vi "createNewExcelDocument.vi"(8 "error in (no error)":errorcluster, 10 "Excel File Path":path, 11 "workbook in":refnum<class "workbook.lvclass">) -> (0 "error out":errorcluster, 3 "workbook out":refnum<class "workbook.lvclass">)   [LabVIEW 2017, in "Excel_Specific.lvlib" / "workbook.lvclass"]
uses:
  workbook.lvclass
  C:/Users/Neo/Desktop/Dev_Tools_BR/LabVIEW_NPOI/src/lib/NPOI 2.1.1/NPOI.OOXML.dll
  lib/NPOI 2.1.1/NPOI.OOXML.dll
  workbook.lvclass/workbook.ctl
  worksheet/worksheet.lvclass
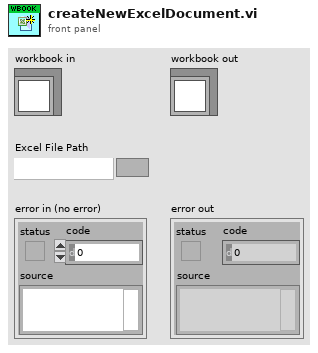
[diagram p1: front panel]
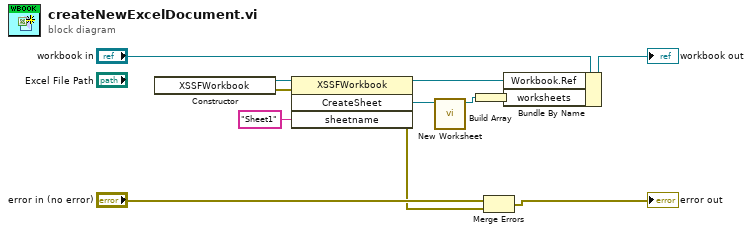
[diagram p0: block diagram]
diagram:
  n1 = constructor class="XSSFWorkbook"() -> (reference out=w9:refnum<k24>, error out=w10:errorcluster)  [unwired: 3 in, 1 out]
  n2 = invoke class="XSSFWorkbook" method="CreateSheet"(reference=w9, error in=w10, "sheetname"="Sheet1") -> (reference out=w6:refnum<k24>, error out=w4:errorcluster, "CreateSheet"=w3:refnum<k24>)  [unwired: 1 in, 1 out]
  n3 = call "New Worksheet.vi"("Worksheet.Ref"=w3) -> ("worksheet out"=w2:refnum<class "worksheet.lvclass">)  [unwired: 9 in, 1 out]
  n4 = Build Array(w2) -> (w1:refnum<class "worksheet.lvclass">[])
  n5 = Merge Errors("error in (no error)", w4) -> (→"error out":errorcluster)
  n6 = Bundle By Name(cluster="workbook in", "Workbook.Ref"=w6, "worksheets"=w1) -> (→"workbook out":refnum<class "workbook.lvclass">)
